vi "Practica 12.vi"() -> ()   [LabVIEW 2018]
uses:
  <vilib>/LabVIEW Interface for Arduino/Type Defs/Digital Pin.ctl
  <vilib>/LabVIEW Interface for Arduino/Type Defs/Pin Mode.ctl
  <vilib>/LabVIEW Interface for Arduino/LabVIEW Interface for Arduino.lvlib
panel:
  out "Estado de salida":bool
  in  "SELECCION DE PUERTO":refnum<visa-resource-name>
  in  "Detener":bool
  in  "ACTIVA/DESACTIVA":bool
  in  "Seleccion de PIN":T1
  # "Practica 12: CONTROL DE SALIDA SELECCIONADA"
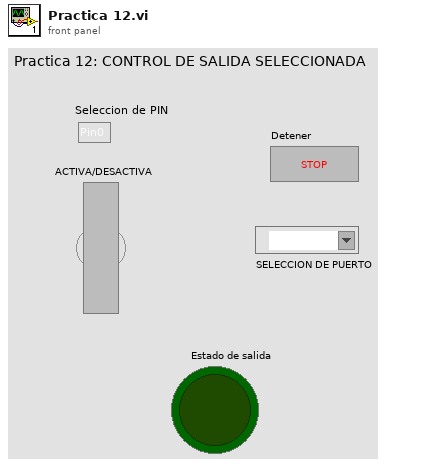
[diagram p1: front panel]
types:
  T1 = typedef "LabVIEW Interface for Arduino.lvlib/Digital Pin.ctl" = enum8{"Pin0", "Pin1", "Pin2", "Pin3", "Pin4", "Pin5", "Pin6", "Pin7", "Pin8", "Pin9", "Pin10", "Pin11", "Pin12", "Pin13"}
  T2 = typedef "LabVIEW Interface for Arduino.lvlib/Arduino Resource.ctl" = cluster{"VISA resource":refnum<visa-resource-name>, "Board Type":T3, "Connection Type":enum8{"USB / Serial"}, "Bytes Per Packet (15)":u8}
  T3 = typedef "LabVIEW Interface for Arduino.lvlib/Board Type.ctl" = enum16{"Uno", "Dimuelanove w/Atmega 328", "Mega 2560"}
  T4 = typedef "LabVIEW Interface for Arduino.lvlib/Pin Mode.ctl" = enum8{"Input", "Output"}
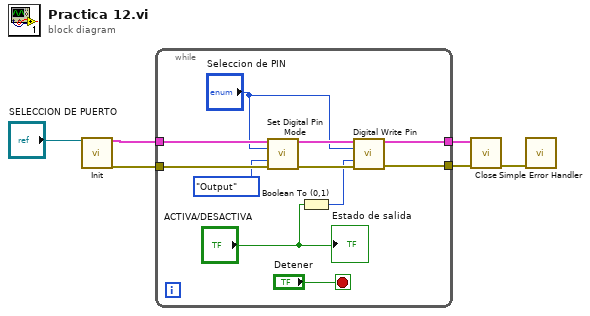
[diagram p0: block diagram]
diagram:
  n1 = call <vilib>:"Init.vi"("VISA resource"="SELECCION DE PUERTO") -> ("Arduino Resource"=w5:T2, "error out"=w4:errorcluster)  [unwired: 17 in]
  n2 = while {
    tunnel: w5 -> [w16]
    tunnel: w4 -> [w15]
    tunnel: [w8] -> w3
    tunnel: [w7] -> w2
    stop <- "Detener" stop-if-true
    n3 = call <vilib>:"Set Digital Pin Mode.vi"("Arduino Resource"=w16, "Digital I/O Pin"="Seleccion de PIN", "Pin Mode (Input)"=Pin_Mode."Output", "error in"=w15) -> ("Arduino Resource"=w13:T2, "error out"=w12:errorcluster)  [unwired: 10 in]
    n4 = Boolean To (0,1)(Boolean="ACTIVA/DESACTIVA") -> (0, 1=w10:i16)
    n5 = call <vilib>:"Digital Write Pin.vi"("Arduino Resource"=w13, "Digital I/O Pin (0)"="Seleccion de PIN", "Value (0)"=w10, "error in"=w12) -> ("Arduino Resource"=w8:T2, "error out"=w7:errorcluster)  [unwired: 10 in]
    "Estado de salida" <- "ACTIVA/DESACTIVA"
  }
  n6 = call <vilib>:"Close.vi"("Arduino Resource"=w3, "error in"=w2) -> ("error out"=w1:errorcluster)  [unwired: 13 in]
  n7 = call <vilib>:"Simple Error Handler.vi"("error in (no error)"=w1) -> ()  [unwired: 4 in, 5 out]
